vi "Flip and Pad for Picture Control.vi"(3 "bmp to LV? (T)":bool=TRUE, 4 "bitmap info":T1, 5 "BMP bitmap":u8[](array[numeric])) -> (2 "picture bitmap":u8[](array[numeric]))   [LabVIEW 2020]
doc: "Transform Windows BMP data to LabVIEW picture bitmap data. Windows gives rows from bottom to top padded out to a 32 bit boundary. LabVIEW expects rows given from top to bottom padded to a 16 bit boundary."
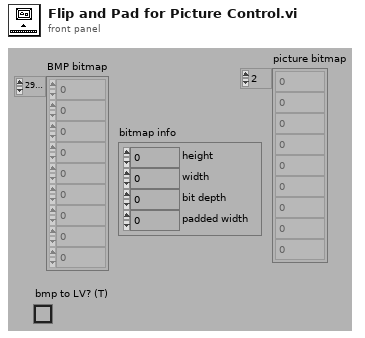
[diagram p1: front panel]
types:
  T1 = cluster{"height":u32, "width":u32, "bit depth":u16, "padded width":u32}
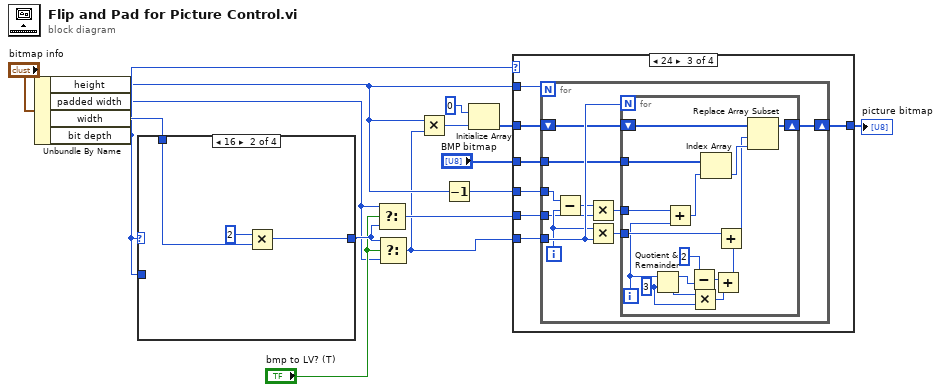
[diagram p0: block diagram]
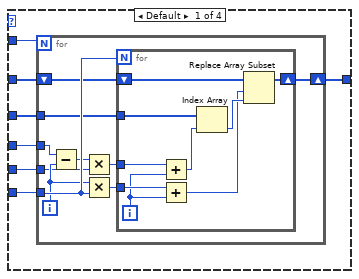
[diagram p2: hidden frame]
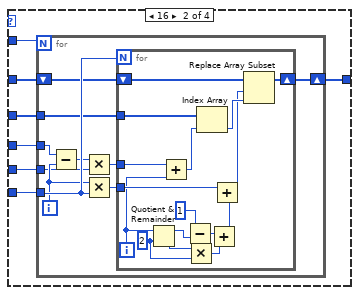
[diagram p3: hidden frame]
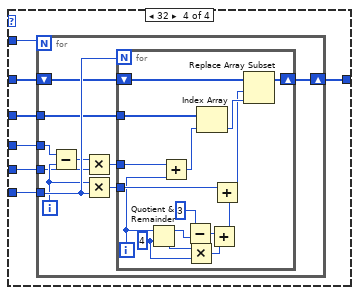
[diagram p4: hidden frame]
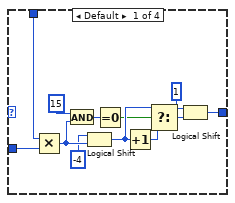
[diagram p5: hidden frame]
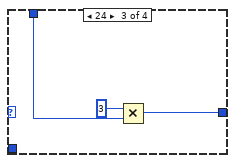
[diagram p6: hidden frame]
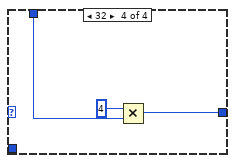
[diagram p7: hidden frame]
diagram:
  n1 = Unbundle By Name("bitmap info") -> ("height"=w4:u32, "padded width"=w2:u32, "width"=w11:u32, "bit depth"=w6:u16)
  n2 = case shown="16" w6 {
    tunnel: w11 -> [w18 w29 w32 w35]
    tunnel: w6 -> [w17 _ _ _]
    tunnel: [w16 w28 w31 w34] -> w9
    frame Default {
      n3 = Multiply(x=w18, y=w17) -> (x*y=w20:u32)
      n4 = And(x=15, y=w20) -> (x .and. y?=w22:u32)
      n5 = Logical Shift(y=-4, x=w20) -> (x << y=w24:u32)
      n6 = Equal To 0?(x=w22) -> (x = 0?=w23:bool)
      n7 = Increment(x=w24) -> (x+1=w25:u32)
      n8 = Select(t=w24, s=w23, f=w25) -> (s? t:f=w27:u32)
      n9 = Logical Shift(y=1, x=w27) -> (x << y=w16:u32)
    }
    frame 16 {
      n10 = Multiply(x=u16 2, y=w29) -> (x*y=w28:u32)
    }
    frame 24 {
      n11 = Multiply(x=u16 3, y=w32) -> (x*y=w31:u32)
    }
    frame 32 {
      n12 = Multiply(x=u16 4, y=w35) -> (x*y=w34:u32)
    }
  }
  n13 = Select(t=w2, s="bmp to LV? (T)", f=w9) -> (s? t:f=w8:u32)
  n14 = Select(t=w9, s="bmp to LV? (T)", f=w2) -> (s? t:f=w1:u32)
  n15 = Multiply(x=w4, y=w1) -> (x*y=w3:u32)
  n16 = Decrement(x=w4) -> (x-1=w15:u32)
  n17 = Initialize Array(u8 0, w3) -> (w14:u8[])
  n18 = case shown="24" w6 {
    tunnel: w15 -> [w43 w69 w102 w135]
    tunnel: w14 -> [w42 w68 w101 w134]
    tunnel: w4 -> [w41 w67 w100 w133]
    tunnel: "BMP bitmap" -> [w40 w66 w99 w132]
    tunnel: w8 -> [w39 w65 w98 w131]
    tunnel: w1 -> [w38 w64 w97 w130]
    tunnel: [w37 w63 w96 w129] -> w5
    frame Default {
      n19 = for {
        N: w41 -> [_]
        shift-right: [w51] -> w37
        shift-left: w42 -> [w52]
        tunnel: w40 -> [w50]
        tunnel: w43 -> [w49]
        tunnel: w39 -> [w44]
        tunnel: w38 -> [w53]
        i -> [w45]
        n20 = Subtract(x=w49, y=w45) -> (x-y=w48:u32)
        n21 = Multiply(x=w48, y=w44) -> (x*y=w47:u32)
        n22 = Multiply(x=w45, y=w53) -> (x*y=w46:u32)
        n23 = for {
          N: w53 -> [_]
          shift-right: [w62] -> w51
          shift-left: w52 -> [w61]
          tunnel: w50 -> [w59]
          tunnel: w47 -> [w58]
          tunnel: w46 -> [w56]
          i -> [w55]
          n24 = Add(x=w58, y=w55) -> (x+y=w57:u32)
          n25 = Add(x=w56, y=w55) -> (x+y=w54:u32)
          n26 = Index Array(array=w59, index=w57) -> (element=w60:u8)
          n27 = Replace Array Subset(array=w61, new element=w60, index=w54) -> (w62:u8[])
        }
      }
    }
    frame 16 {
      n28 = for {
        N: w67 -> [_]
        shift-right: [w77] -> w63
        shift-left: w68 -> [w78]
        tunnel: w66 -> [w76]
        tunnel: w69 -> [w75]
        tunnel: w65 -> [w70]
        tunnel: w64 -> [w79]
        i -> [w71]
        n29 = Subtract(x=w75, y=w71) -> (x-y=w74:u32)
        n30 = Multiply(x=w74, y=w70) -> (x*y=w73:u32)
        n31 = Multiply(x=w71, y=w79) -> (x*y=w72:u32)
        n32 = for {
          N: w79 -> [_]
          shift-right: [w95] -> w77
          shift-left: w78 -> [w94]
          tunnel: w76 -> [w92]
          tunnel: w73 -> [w91]
          tunnel: w72 -> [w89]
          i -> [w87]
          w81 = 2
          n33 = Quotient & Remainder(x=w87, y=w81) -> (x-y*floor(x/y)=w85:i32, floor(x/y)=w82:i32)
          n34 = Add(x=w91, y=w87) -> (x+y=w90:u32)
          n35 = Subtract(x=1, y=w85) -> (x-y=w84:i32)
          n36 = Multiply(x=w82, y=w81) -> (x*y=w80:i32)
          n37 = Index Array(array=w92, index=w90) -> (element=w93:u8)
          n38 = Add(x=w84, y=w80) -> (x+y=w83:i32)
          n39 = Add(x=w89, y=w83) -> (x+y=w88:u32)
          n40 = Replace Array Subset(array=w94, new element=w93, index=w88) -> (w95:u8[])
        }
      }
    }
    frame 24 {
      n41 = for {
        N: w100 -> [_]
        shift-right: [w110] -> w96
        shift-left: w101 -> [w111]
        tunnel: w99 -> [w109]
        tunnel: w102 -> [w108]
        tunnel: w98 -> [w103]
        tunnel: w97 -> [w112]
        i -> [w104]
        n42 = Subtract(x=w108, y=w104) -> (x-y=w107:u32)
        n43 = Multiply(x=w107, y=w103) -> (x*y=w106:u32)
        n44 = Multiply(x=w104, y=w112) -> (x*y=w105:u32)
        n45 = for {
          N: w112 -> [_]
          shift-right: [w128] -> w110
          shift-left: w111 -> [w127]
          tunnel: w109 -> [w125]
          tunnel: w106 -> [w124]
          tunnel: w105 -> [w122]
          i -> [w120]
          w114 = 3
          n46 = Quotient & Remainder(x=w120, y=w114) -> (x-y*floor(x/y)=w118:i32, floor(x/y)=w115:i32)
          n47 = Add(x=w124, y=w120) -> (x+y=w123:u32)
          n48 = Subtract(x=2, y=w118) -> (x-y=w117:i32)
          n49 = Multiply(x=w115, y=w114) -> (x*y=w113:i32)
          n50 = Index Array(array=w125, index=w123) -> (element=w126:u8)
          n51 = Add(x=w117, y=w113) -> (x+y=w116:i32)
          n52 = Add(x=w122, y=w116) -> (x+y=w121:u32)
          n53 = Replace Array Subset(array=w127, new element=w126, index=w121) -> (w128:u8[])
        }
      }
    }
    frame 32 {
      n54 = for {
        N: w133 -> [_]
        shift-right: [w143] -> w129
        shift-left: w134 -> [w144]
        tunnel: w132 -> [w142]
        tunnel: w135 -> [w141]
        tunnel: w131 -> [w136]
        tunnel: w130 -> [w145]
        i -> [w137]
        n55 = Subtract(x=w141, y=w137) -> (x-y=w140:u32)
        n56 = Multiply(x=w140, y=w136) -> (x*y=w139:u32)
        n57 = Multiply(x=w137, y=w145) -> (x*y=w138:u32)
        n58 = for {
          N: w145 -> [_]
          shift-right: [w161] -> w143
          shift-left: w144 -> [w160]
          tunnel: w142 -> [w158]
          tunnel: w139 -> [w157]
          tunnel: w138 -> [w155]
          i -> [w153]
          w147 = 4
          n59 = Quotient & Remainder(x=w153, y=w147) -> (x-y*floor(x/y)=w151:i32, floor(x/y)=w148:i32)
          n60 = Add(x=w157, y=w153) -> (x+y=w156:u32)
          n61 = Subtract(x=3, y=w151) -> (x-y=w150:i32)
          n62 = Multiply(x=w148, y=w147) -> (x*y=w146:i32)
          n63 = Index Array(array=w158, index=w156) -> (element=w159:u8)
          n64 = Add(x=w150, y=w146) -> (x+y=w149:i32)
          n65 = Add(x=w155, y=w149) -> (x+y=w154:u32)
          n66 = Replace Array Subset(array=w160, new element=w159, index=w154) -> (w161:u8[])
        }
      }
    }
  }
  "picture bitmap" <- w5
